vi "add data to plot 2.vi"(0 "Current":dbl[](array[numeric]), 1 "Voltage":dbl[](array[numeric]), 3 "Voltage targets":dbl[](array[numeric]), 5 "error in (no error)":errorcluster, 6 "i":dbl, 7 "t0":dbl, 10 "v":dbl, 11 "dt":dbl, 12 "voltage target":dbl) -> (14 "Current cluster":cluster{"t0":dbl, "dt":dbl, "Current":dbl[]}, 15 "Voltage graph":cluster{"t0":dbl, "dt":dbl, dbl[][]}, 16 "output current":dbl[](array[numeric]), 17 "output voltage":dbl[](array[numeric]), 18 "Voltage target":dbl[](array[numeric]), 19 "error in (no error) 2":errorcluster)   [LabVIEW 2020]
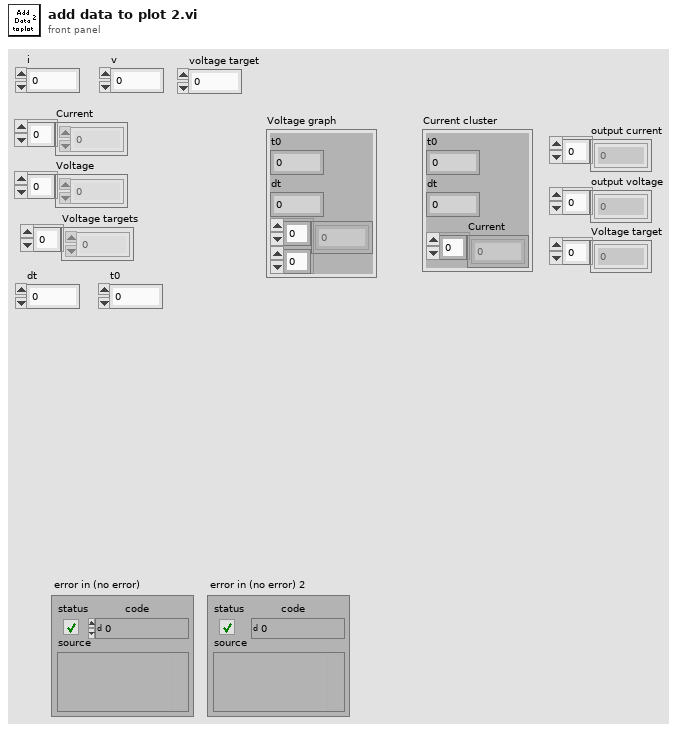
[diagram p1: front panel]
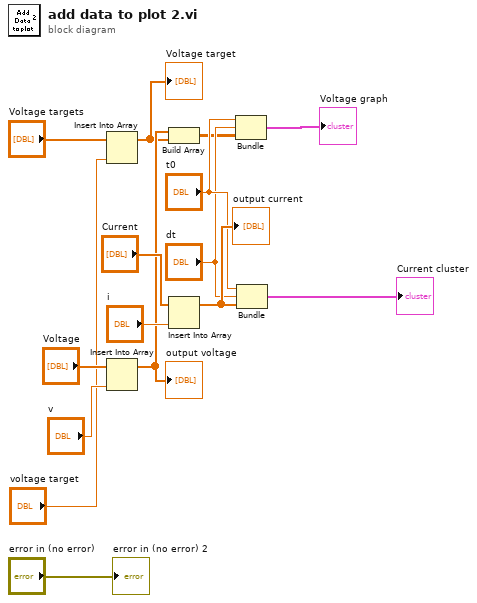
[diagram p0: block diagram]
diagram:
  n1 = Insert Into Array(array="Voltage targets", new element="voltage target") -> (w7:dbl[])  [unwired: 1 in]
  "Voltage target" <- w7
  n2 = Insert Into Array(array="Voltage", new element="v") -> (w10:dbl[])  [unwired: 1 in]
  "output voltage" <- w10
  n3 = Build Array(w10, w7) -> (w3:dbl[][])
  n4 = Insert Into Array(array="Current", new element="i") -> (w6:dbl[])  [unwired: 1 in]
  "output current" <- w6
  n5 = Bundle("t0"="t0", "dt"="dt", w3) -> (→"Voltage graph":cluster{"t0":dbl, "dt":dbl, dbl[][]})  [unwired: 1 in]
  n6 = Bundle("t0"="t0", "dt"="dt", "Current"=w6) -> (→"Current cluster":cluster{"t0":dbl, "dt":dbl, "Current":dbl[]})  [unwired: 1 in]
  "error in (no error) 2" <- "error in (no error)"
